vi "Initialise.vi"(8 "error in (no error)":errorcluster, 11 "OpenSSL Client Context in":refnum<class "SSL Client Context.lvclass">) -> (0 "error out":errorcluster, 3 "OpenSSL Client Context out":refnum<class "SSL Client Context.lvclass">)   [LabVIEW 2013, in "OpenSSL Socket.lvlib" / "SSL Client Context.lvclass"]
uses:
  SSL Client Context.lvclass
  SSL_Lib/SSL-Context/SSL Verify Mode.ctl
  SSL Context/SSL Context.lvclass/SSL Context.ctl
  SSL Client Context.lvclass/SSL Client Context.ctl
  SSL Context/Read SSL Context.vi
  Read SSL Options.vi
  Read Cipher List.vi
  Read Verification Options.vi
  Read Verification Depth.vi
  Read Verification CA Bundle Path.vi
  SSL_Lib/SSL-Context/SSL-Context.lvclass
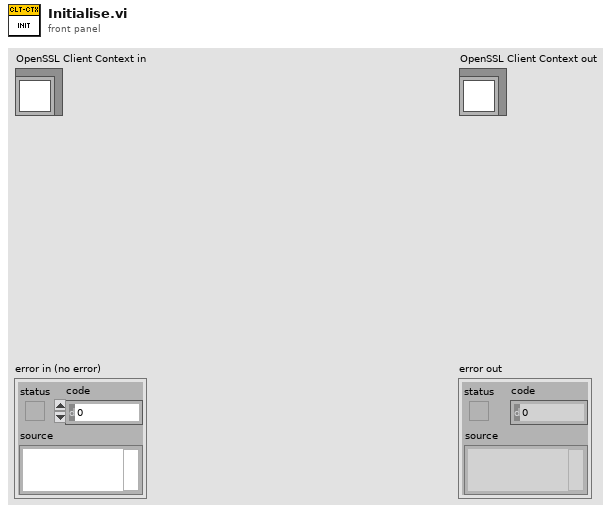
[diagram p1: front panel]
types:
  T1 = typedef "SSL_Lib.lvlib/SSL-Context.lvclass/SSL Verify Mode.ctl" = i32
  T2 = typedef "SSL_Lib.lvlib/SSL-Context.lvclass/SSL Options.ctl" = i32
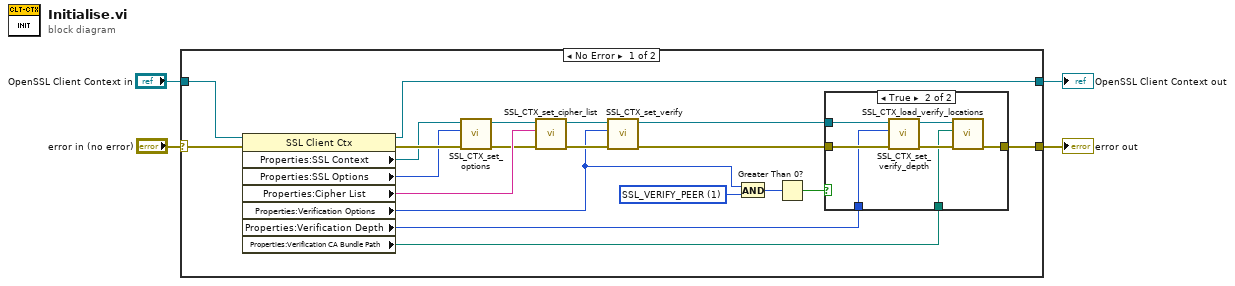
[diagram p0: block diagram]
diagram:
  n1 = case shown="No Error" "error in (no error)" {
    selector: "error in (no error)" -> [w6 w34]
    tunnel: "OpenSSL Client Context in" -> [w24 w33]
    tunnel: [w10 w33] -> w3
    tunnel: [w7 w34] -> w2
    frame No Error {
      w15 = T1 1 items=["SSL_VERIFY_PEER|FAIL_IF_NO_PEER_CERT"=3, "SSL_VERIFY_NONE"=0, "SSL_VERIFY_PEER"=1, "SSL_VERIFY_FAIL_IF_NO_PEER_CERT"=2, "SSL_VERIFY_CLIENT_ONCE"=4] ("Mode")
      n2 = property class="SSL Client Ctx"(reference=w24, error in=w6) -> (reference out=w10:refnum<class "SSL Client Context.lvclass">, error out=w23:errorcluster, "Properties:SSL Context"=w20:refnum<class "SSL-Context.lvclass">, "Properties:SSL Options"=w22:T2, "Properties:Cipher List"=w21:string, "Properties:Verification Options"=w14:T1, "Properties:Verification Depth"=w9:i32, "Properties:Verification CA Bundle Path"=w8:path)
      n3 = call "SSL_CTX_set_options.vi"("error in (no error)"=w23, "Options"=w22, "SSL-Context in"=w20) -> ("error out"=w19:errorcluster, "SSL-Context out"=w18:refnum<class "SSL-Context.lvclass">)  [unwired: 7 in]
      n4 = call "SSL_CTX_set_cipher_list.vi"("error in (no error)"=w19, "Cipher List"=w21, "SSL-Context in"=w18) -> ("error out"=w17:errorcluster, "SSL-Context out"=w16:refnum<class "SSL-Context.lvclass">)  [unwired: 7 in]
      n5 = call "SSL_CTX_set_verify.vi"("error in (no error)"=w17, "Mode"=w14, "SSL-Context in"=w16) -> ("error out"=w12:errorcluster, "SSL-Context out"=w11:refnum<class "SSL-Context.lvclass">)  [unwired: 7 in]
      n6 = And(x=w14, y=w15) -> (x .and. y?=w13:T1)
      n7 = Greater Than 0?(x=w13) -> (x > 0?=w5:bool)
      n8 = case shown="True" w5 {
        tunnel: w12 -> [w25 w32]
        tunnel: w11 -> [_ w31]
        tunnel: w9 -> [_ w28]
        tunnel: w8 -> [_ w27]
        tunnel: [w25 w26] -> w7
        frame False {
        }
        frame True {
          n9 = call "SSL_CTX_set_verify_depth.vi"("error in (no error)"=w32, "Depth"=w28, "SSL-Context in"=w31) -> ("error out"=w29:errorcluster, "SSL-Context out"=w30:refnum<class "SSL-Context.lvclass">)  [unwired: 7 in]
          n10 = call "SSL_CTX_load_verify_locations.vi"("error in (no error)"=w29, "Path to CA bundle"=w27, "SSL-Context in"=w30) -> ("error out"=w26:errorcluster)  [unwired: 7 in, 1 out]
        }
      }
    }
    frame Error {
    }
  }
  "error out" <- w2
  "OpenSSL Client Context out" <- w3
